vi "IP V1.vi"(0 "Image In":T1, 5 "Image Dst":T1, 7 "BinImage":T1, 9 "Zoom Image":T1, 12 "error in":errorcluster) -> (2 "Threshold Range Out":cluster{"Lower value":sgl, "Upper value":sgl}={"Lower value"=128.0, "Upper value"=255.0} {"Upper value" format="%.2f"; "Lower value" format="%.2f"}, 3 "VerCenter":u32, 6 "MaxA":u32, 8 "MaxB":u32, 10 "HorCenter":u16, 13 "output cluster":T2, 14 "MaxY":u32, 15 "MaxX":u32)   [LabVIEW 2015]
doc: "Creates, edits, and runs vision algorithms using NI Vision Assistant.\n\nWhen you place this Express VI on the block diagram, NI Vision Assistant launches. Create an algorithm using the Vision Assistant processing functions. After you create an algorithm, you can select the controls and indicators that you want to be able to programmatically set in LabVIEW. Double-click the Vision Assistant Express VI to edit the algorithm."
uses:
  <vilib>/vision/Image Controls.llb/IMAQ Image.ctl
  Controls/Pivot Finder Input Params Typedef.ctl
  <vilib>/vision/NI_Vision_Development_Module.lvlib
panel:
  out "CtualThresh":cluster{"Lower value":sgl, "Upper value":sgl}
  in  "CircleQualityThrs":dbl=1.0
  in  "AutoRange":bool
  in  "RangeGain":sgl=5e-05 format="%#.8f"
  in  "StartRadius":u16=150
  in  "EndRadius":u16=200
  out "MaxGrade":u32
  out "Image Dst Out":T1(plugin-control)
  out "Sum 2":u8[][](graph)
  out "transposed array":u8[][](graph)
  in  "Threshold Limits":cluster{"Lower value":sgl, "Upper value":sgl}={"Lower value"=0.0, "Upper value"=255.0} {"Upper value" format="%.2f"; "Lower value" format="%.2f"}
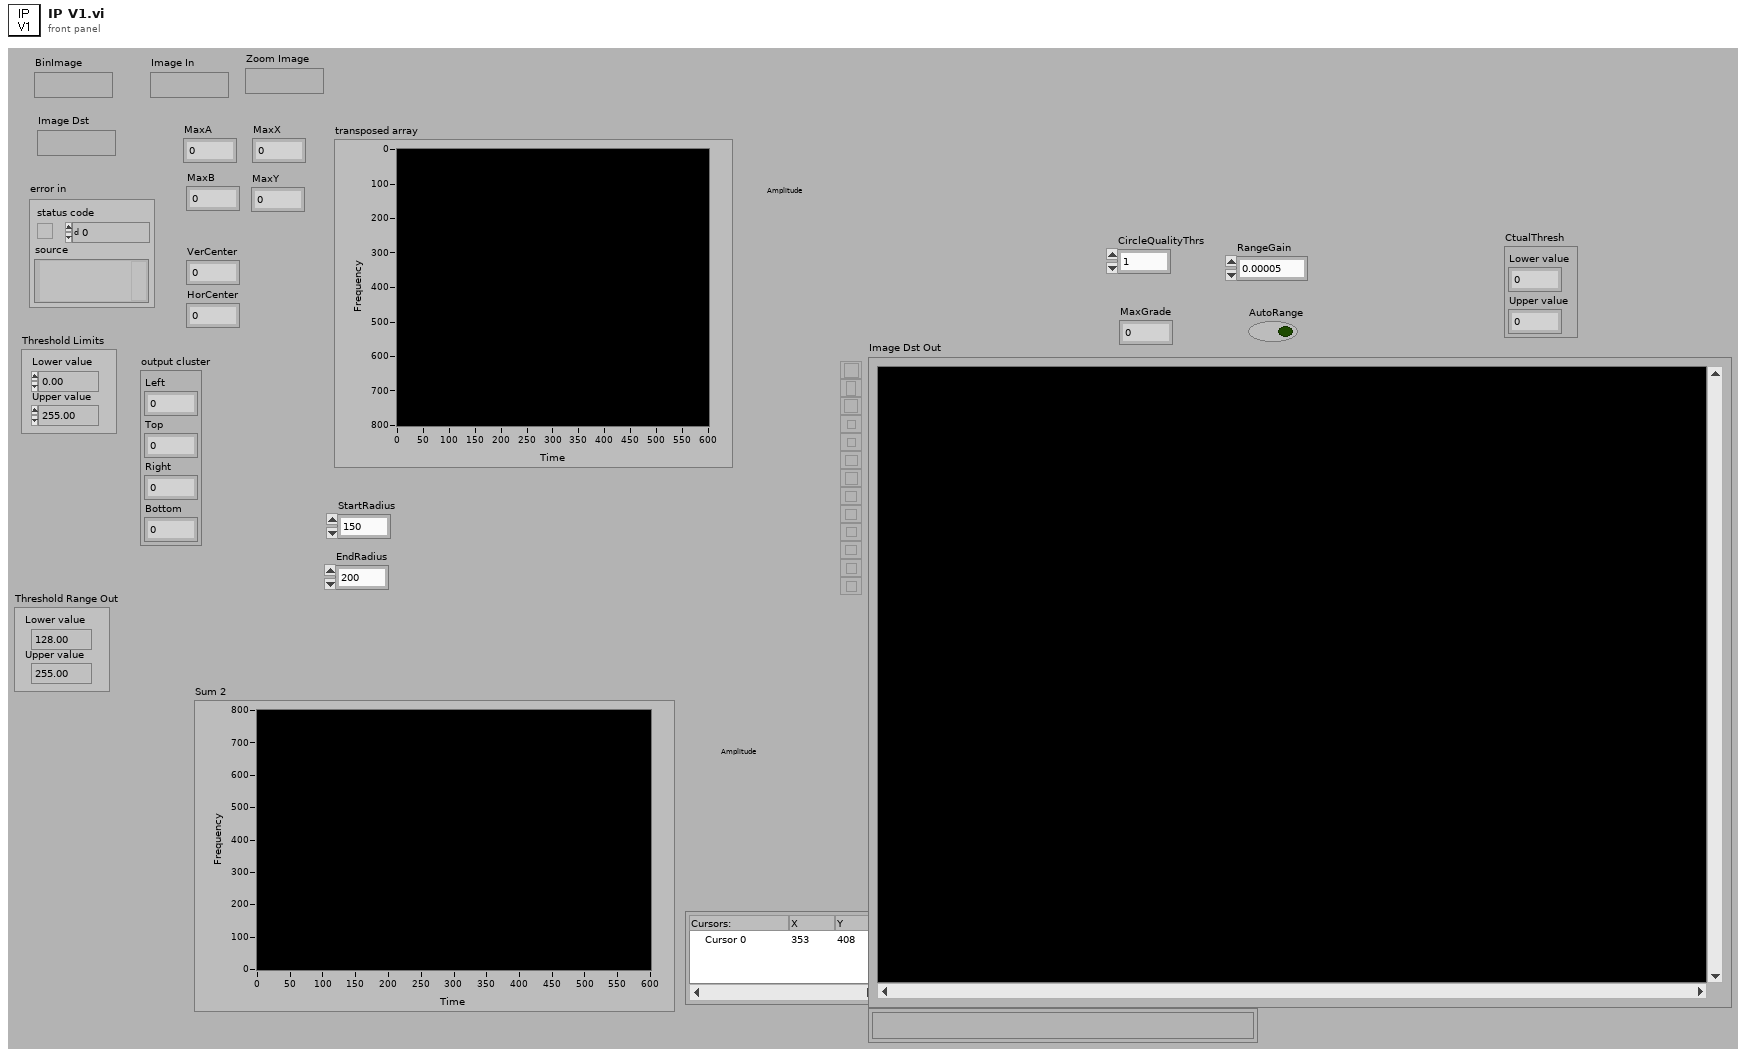
[diagram p1: front panel]
types:
  T1 = typedef "IMAQ Image.ctl" = refnum<image>
  T2 = cluster{"Left":i32, "Top":i32, "Right":i32, "Bottom":i32}
  T3 = typedef "Pivot Finder Input Params Typedef.ctl" = cluster{"Ymin":u32, "Ymax":u32, "Xmin":u32, "Xmax":u32, "Amin":u32, "Amax":u32, "Bmin":u32, "Bmax":u32}
  T4 = cluster{"Ymin":dbl, "Ymax":dbl, "Xmin":dbl, "Xmax":dbl, "Amin":dbl, "Amax":dbl, "Bmin":dbl, "Bmax":dbl}
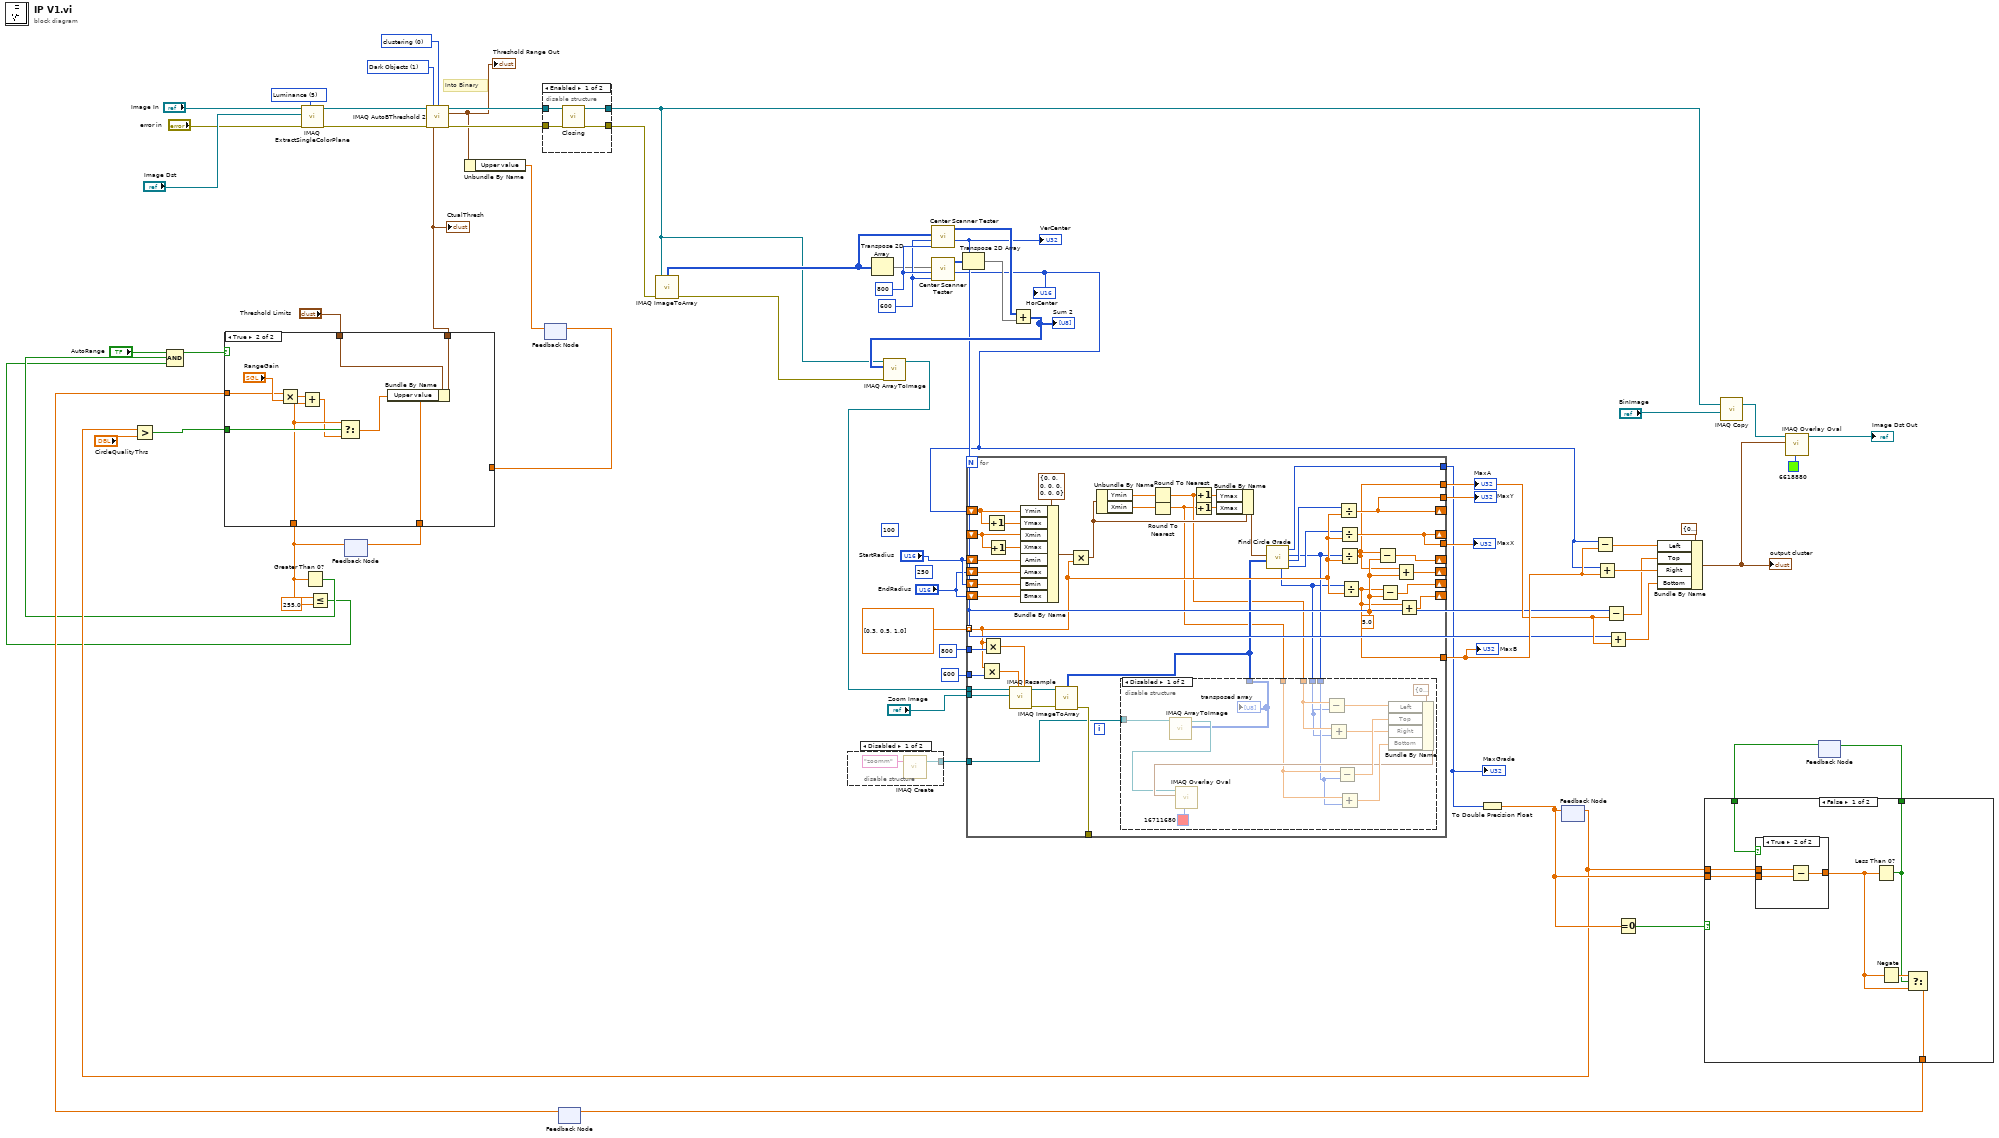
[diagram p0: block diagram]
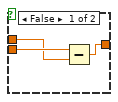
[diagram p4: hidden frame]
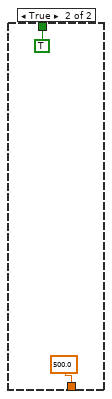
[diagram p5: hidden frame]
diagram:
  w56 = u16 800 ("Hight")
  w55 = u16 600 ("Width")
  (unwired) u16 250 ("Amin")
  (unwired) u16 100 ("Amin")
  w65 = u32 1 items=["Bright Objects", "Dark Objects"] ("Look For (Bright Objects)")
  w66 = 0 items=["clustering", "entropy", "metric", "moments", "inter-class variance"] ("Method")
  w67 = 5 items=["Red", "Green", "Blue", "Hue", "Saturation", "Luminance", "Value", "Intensity"] ("Color Plane")
  # "Into Binary"
  n1 = call "IMAQ ExtractSingleColorPlane"("Color Plane"=w67, "error in (no error)"="error in", "Image Dst"="Image Dst", "Image Src"="Image In") -> ("error out"=w41:errorcluster, "Image Dst Out"=w40:T1)  [unwired: 6 out]
  n2 = feedback #1() -> (w3:dbl)  [unwired: 1 in]
  n3 = Greater Than 0?(x=w3) -> (x > 0?=w4:bool)
  n4 = Less Or Equal?(x=w3, y=255.0) -> (x <= y?=w1:bool)
  n5 = Compound Arithmetic op=AND("AutoRange", w4, w1) -> (w5:bool)
  n6 = feedback #2() -> (w7:sgl)  [unwired: 1 in]
  n7 = feedback #3() -> (w16:dbl)  [unwired: 1 in]
  n8 = disable-structure shown="Disabled" {
    disable-tunnel: [w68 _] -> w37
    frame Disabled {
      n9 = call "IMAQ Create"("Image Name"="zoomm") -> ("New Image"=w68:T1)  [unwired: 3 in, 2 out]
    }
    frame Enabled {
    }
  }
  n10 = feedback #4() -> (w10:dbl)  [unwired: 1 in]
  n11 = Greater?(x=w10, y="CircleQualityThrs") -> (0:w9:bool)
  n12 = case shown="True" w5 {
    tunnel: "Threshold Limits" -> [w71 w80]
    tunnel: [w71 w79] -> w18
    tunnel: [w70 w75] -> w21
    tunnel: w3 -> [_ w73]
    tunnel: w9 -> [_ w76]
    tunnel: w16 -> [_ w74]
    tunnel: w7 -> [w70 _]
    frame False {
    }
    frame True {
      n13 = Multiply(x=w74, y="RangeGain") -> (x*y=w77:dbl)
      n14 = Add(x=w77, y=w73) -> (x+y=w72:dbl)
      n15 = Select(t=w73, s=w76, f=w72) -> (s? t:f=w75:dbl)
      n16 = Bundle By Name(cluster=w80, "Upper value"=w75) -> (w79:cluster{"Lower value":sgl, "Upper value":sgl})
    }
  }
  "CtualThresh" <- w18
  n17 = feedback-in #1(w21) -> ()
  n18 = call "IMAQ AutoBThreshold 2"("Image Src"=w40, "Look For (Bright Objects)"=w65, "Method (clustering)"=w66, "error in (no error)"=w41, "Threshold Limits"=w18) -> ("Image Dst Out"=w51:T1, "Threshold Range Out"=w14:cluster{"Lower value":sgl, "Upper value":sgl}, "error out"=w50:errorcluster)  [unwired: 3 in, 5 out]
  "Threshold Range Out" <- w14
  n19 = Unbundle By Name(w14) -> ("Upper value"=w8:sgl)
  n20 = disable-structure shown="Enabled" {
    disable-tunnel: [w84 w85] -> w64
    disable-tunnel: w51 -> [w83 w86]
    disable-tunnel: w50 -> [w82 w85]
    disable-tunnel: [w81 w86] -> w32
    frame Enabled {
      n21 = call "Closing.vi"("error in (no error)"=w82, "Refnum in"=w83) -> ("error out"=w84:errorcluster, "Refnum out"=w81:T1)  [unwired: 8 in]
    }
    frame Disabled {
    }
  }
  n22 = feedback-in #2(w8) -> ()
  n23 = call "IMAQ ImageToArray"("error in (no error)"=w64, "Image"=w32) -> ("error out"=w31:errorcluster, "Image Pixels (U8)"=w54:u8[][])  [unwired: 2 in, 3 out]
  n24 = Transpose 2D Array(2D array=w54) -> (transposed array=w53:u8[][])
  n25 = call "Center Scanner Tester.vi"("Hight"=w56, "Width"=w55, "ImageIn"=w54) -> ("HorCenter"=w34:u16, "ImgOut"=w47:u8[][])  [unwired: 7 in]
  "VerCenter" <- w34
  n26 = call "Center Scanner Tester.vi"("Hight"=w55, "Width"=w56, "ImageIn"=w53) -> ("HorCenter"=w33:u16, "ImgOut"=w46:u8[][])  [unwired: 7 in]
  "HorCenter" <- w33
  n27 = Transpose 2D Array(2D array=w46) -> (transposed array=w45:u8[][])
  n28 = Add(x=w47, y=w45) -> (x+y=w39:u8[][])
  "Sum 2" <- w39
  n29 = call "IMAQ ArrayToImage"("error in (no error)"=w31, "Image Pixels (U8)"=w39, "Image"=w32) -> ("Image Out"=w38:T1)  [unwired: 7 in, 1 out]
  n30 = for {
    tunnel: "Zoom Image" -> [w128]
    tunnel: w38 -> [w129]
    tunnel: dbl[] [0.3, 0.5, 1.0] -> [w116] mode=indexing
    tunnel: 800 -> [w127]
    tunnel: 600 -> [w126]
    shift-right: [w100] -> _
    shift-left: w33 -> [w120]
    shift-right: [w99] -> _
    shift-left: w34 -> [w119]
    shift-right: [w112] -> _
    shift-left: "StartRadius" -> [w115]
    shift-right: [w111] -> _
    shift-left: "EndRadius" -> [w118]
    shift-right: [w108] -> _
    shift-left: "StartRadius" -> [w114]
    shift-right: [w110] -> _
    shift-left: "EndRadius" -> [w113]
    tunnel: [w107] -> _
    tunnel: [w96] -> w36
    tunnel: [w99] -> w48
    tunnel: [w97] -> w35
    tunnel: [w100] -> w49
    tunnel: w37 -> [w93]
    tunnel: [w87] -> w22
    w109 = 5.0 ("y")
    n31 = Multiply(x=w116, y=w126) -> (x*y=w125:dbl)
    n32 = Multiply(x=w116, y=w127) -> (x*y=w124:dbl)
    n33 = Increment(x=w120) -> (x+1=w123:dbl)
    n34 = Increment(x=w119) -> (x+1=w122:dbl)
    n35 = call "IMAQ Resample"("X Resolution"=w124, "Y Resolution"=w125, "Image Dst"=w128, "Image Src"=w129) -> ("error out"=w130:errorcluster, "Image Dst Out"=w95:T1)  [unwired: 6 in]
    n36 = Bundle By Name(cluster=T3 {"Ymin"=0, "Ymax"=0, "Xmin"=0, "Xmax"=0, "Amin"=0, "Amax"=0, "Bmin"=0, "Bmax"=0} ("Cluster"), "Ymin"=w120, "Ymax"=w123, "Xmin"=w119, "Xmax"=w122, "Amin"=w115, "Amax"=w118, "Bmin"=w114, "Bmax"=w113) -> (w117:T3)
    n37 = call "IMAQ ImageToArray"("error in (no error)"=w130, "Image"=w95) -> ("error out"=w107:errorcluster, "Image Pixels (U8)"=w92:u8[][])  [unwired: 2 in, 3 out]
    n38 = Multiply(x=w117, y=w116) -> (x*y=w103:T4)
    n39 = Unbundle By Name(w103) -> ("Ymin"=w94:dbl, "Xmin"=w98:dbl)
    n40 = Round To Nearest(number=w94) -> (nearest integer value=w91:dbl)
    n41 = Round To Nearest(number=w98) -> (nearest integer value=w90:dbl)
    n42 = Increment(x=w91) -> (x+1=w105:dbl)
    n43 = Increment(x=w90) -> (x+1=w104:dbl)
    n44 = Bundle By Name(cluster=w103, "Ymax"=w105, "Xmax"=w104) -> (w106:T4)
    n45 = call "Find Circle Grade.vi"("Picture"=w92, "Cluster"=w106) -> ("MaxX"=w102:u32, "MaxY"=w101:u32, "MaxA"=w89:u32, "MaxGrade"=w87:u32, "MaxB"=w88:u32)  [unwired: 5 in]
    n46 = disable-structure shown="Disabled" {
      disable-tunnel: w93 -> [w137 _]
      disable-tunnel: w92 -> [w135 _]
      disable-tunnel: w91 -> [w134 _]
      disable-tunnel: w90 -> [w133 _]
      disable-tunnel: w89 -> [w132 _]
      disable-tunnel: w88 -> [w131 _]
      frame Disabled {
        n47 = call "IMAQ ArrayToImage"("Image Pixels (U8)"=w135, "Image"=w137) -> ("Image Out"=w136:T1)  [unwired: 8 in, 1 out]
        n48 = Subtract(x=w134, y=w131) -> (x-y=w141:dbl)
        n49 = Add(x=w134, y=w131) -> (x+y=w142:dbl)
        n50 = Subtract(x=w133, y=w132) -> (x-y=w143:dbl)
        n51 = Add(x=w133, y=w132) -> (x+y=w144:dbl)
        n52 = Bundle By Name(cluster=T2 {"Left"=0, "Top"=0, "Right"=0, "Bottom"=0} ("Bounding Rectangle"), "Left"=w141, "Top"=w143, "Right"=w142, "Bottom"=w144) -> (w138:T2)
        n53 = call "IMAQ Overlay Oval"("Color"=u32 16711680, "Bounding Rectangle"=w138, "Image"=w136) -> ()  [unwired: 7 in, 2 out]
        "transposed array" <- w135
      }
      frame Enabled {
      }
    }
    n54 = Divide(x=w101, y=w116) -> (x/y=w100:dbl)
    n55 = Divide(x=w102, y=w116) -> (x/y=w99:dbl)
    n56 = Divide(x=w89, y=w116) -> (x/y=w97:dbl)
    n57 = Divide(x=w88, y=w116) -> (x/y=w96:dbl)
    n58 = Subtract(x=w97, y=w109) -> (x-y=w112:dbl)
    n59 = Subtract(x=w96, y=w109) -> (x-y=w108:dbl)
    n60 = Add(x=w97, y=w109) -> (x+y=w111:dbl)
    n61 = Add(x=w96, y=w109) -> (x+y=w110:dbl)
  }
  "MaxA" <- w35
  "MaxY" <- w49
  "MaxX" <- w48
  "MaxB" <- w36
  "MaxGrade" <- w22
  n62 = To Double Precision Float(number=w22) -> (double precision float=w15:dbl)
  n63 = feedback-in #4(w15) -> ()
  n64 = Subtract(x=w33, y=w36) -> (x-y=w60:dbl)
  n65 = Add(x=w33, y=w36) -> (x+y=w59:dbl)
  n66 = Subtract(x=w34, y=w35) -> (x-y=w58:dbl)
  n67 = Add(x=w34, y=w35) -> (x+y=w57:dbl)
  n68 = Equal To 0?(x=w15) -> (x = 0?=w13:bool)
  n69 = Bundle By Name(cluster=T2 {"Left"=0, "Top"=0, "Right"=0, "Bottom"=0} ("Bounding Rectangle"), "Left"=w60, "Top"=w58, "Right"=w59, "Bottom"=w57) -> (w25:T2)
  "output cluster" <- w25
  n70 = call "IMAQ Copy"("Image Dst"="BinImage", "Image Src"=w32) -> ("Image Dst Out"=w28:T1)  [unwired: 1 in, 4 out]
  n71 = call "IMAQ Overlay Oval"("Color"=u32 6618880, "Bounding Rectangle"=w25, "Image"=w28) -> ("Image Out"=→"Image Dst Out":T1)  [unwired: 7 in, 1 out]
  n72 = feedback #5() -> (w11:bool)  [unwired: 1 in]
  n73 = case shown="False" w13 {
    tunnel: [w147 500.0] -> w17
    tunnel: w10 -> [w150 _]
    tunnel: w15 -> [w149 _]
    tunnel: [w146 TRUE] -> w12
    tunnel: w11 -> [w145 _]
    frame False {
      n74 = case shown="True" w145 {
        tunnel: w150 -> [w152 w157]
        tunnel: w149 -> [w153 w156]
        tunnel: [w154 w155] -> w148
        frame False {
          n75 = Subtract(x=w153, y=w152) -> (x-y=w154:dbl)
        }
        frame True {
          n76 = Subtract(x=w157, y=w156) -> (x-y=w155:dbl)
        }
      }
      n77 = Less Than 0?(x=w148) -> (x < 0?=w146:bool)
      n78 = Negate(x=w148) -> (-x=w151:dbl)
      n79 = Select(t=w151, s=w146, f=w148) -> (s? t:f=w147:dbl)
    }
    frame True {
    }
  }
  n80 = feedback-in #3(w17) -> ()
  n81 = feedback-in #5(w12) -> ()
